vi "ConfigureCurrentRegulator.vi"(0 "axis in":cluster{"keyHandle":u32, "nodeId":u16}={"keyHandle"=0, "nodeId"=1}, 9 "current gains":cluster{"p-Gain":u16, "i-Gain":u16}, 11 "error in (no error)":errorcluster) -> (4 "axis out":cluster{"keyHandle":u32, "nodeId":u16}={"keyHandle"=0, "nodeId"=1}, 15 "error out":errorcluster)   [LabVIEW 2017, in "maxonEPOS.lvlib"]
doc: "<B>ConfigureCurrentRegulator</B> writes the current regulation gain parameters to the device."
uses:
  Examples/maxonEPOS.lvlib
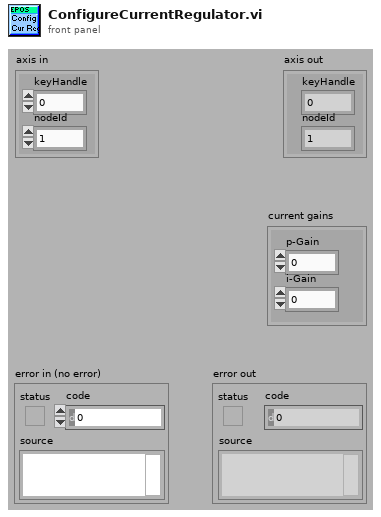
[diagram p1: front panel]
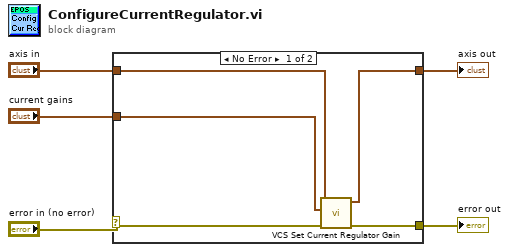
[diagram p0: block diagram]
diagram:
  n1 = case shown="No Error" "error in (no error)" {
    selector: "error in (no error)" -> [w6 w12]
    tunnel: [w10 w12] -> w4
    tunnel: [w9 w11] -> w3
    tunnel: "axis in" -> [w7 w11]
    tunnel: "current gains" -> [w8 _]
    frame No Error {
      n2 = call "VCS Set Current Regulator Gain.vi"("error in (no error)"=w6, "gains"=w8, "axis in"=w7) -> ("error out"=w10:errorcluster, "axis out"=w9:cluster{"keyHandle":u32, "nodeId":u16})  [unwired: 7 in]
    }
    frame Error {
    }
  }
  "error out" <- w4
  "axis out" <- w3
